vi "MK210_Query.vi"(7 "String":string, 8 "error in (no error)":errorcluster, 9 "Delay Time (s) 2":dbl=0.5, 10 "Delay Time (s)":dbl=0.5, 11 "DriverConnect in":T1) -> (0 "error out":errorcluster, 3 "DriverConnect out":T1, 4 "String from device out":string)   [LabVIEW 2018]
uses:
  MOKO_LabViewLibrary/MokoLowLevel/MokoLowLovelControl/MLLC_ConnectCluster.ctl
  MOKO_LabViewLibrary/MokoLowLevel/MokoLowLovelControl/MLLC_InterfaceType.ctl
  MOKO_LabViewLibrary/MokoLowLevel/MokoLowLovelControl/MLLC_OpenedSession.ctl
  MOKO_LabViewLibrary/MokoLowLevel/MokoLowLovelControl/MLLC_InterfaceSettings.ctl
  MOKO_LabViewLibrary/MokoLowLevel/MokoLowLovelControl/MLLC_InterfaceKind.ctl
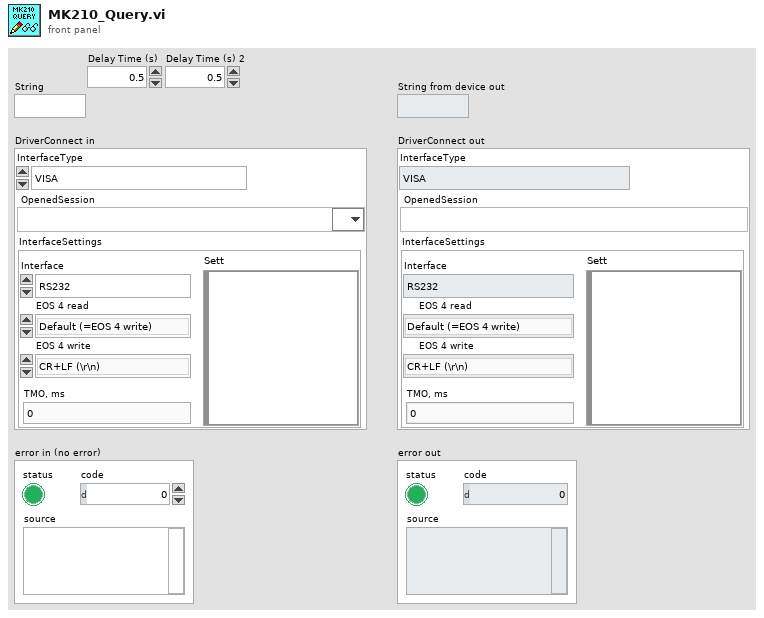
[diagram p1: front panel]
types:
  T1 = typedef "MLLC_ConnectCluster.ctl" = cluster{"InterfaceType":T2, "OpenedSession":T3, "InterfaceSettings":T4}
  T2 = typedef "MLLC_InterfaceType.ctl" = enum16{"VISA", "Prologix USB-GPIB"}
  T3 = typedef "MLLC_OpenedSession.ctl" = refnum<visa-resource-name>
  T4 = typedef "MLLC_InterfaceSettings.ctl" = cluster{"Interface":T5, "EOS 4 read":enum16{"Default (=EOS 4 write)", "CR (\\r)", "LF (\\n)", "None"}, "EOS 4 write":enum16{"CR+LF (\\r\\n)", "CR (\\r)", "LF (\\n)", "None"}, "TMO, ms":i32, "Sett":variant}
  T5 = typedef "MLLC_InterfaceKind.ctl" = enum16{"RS232", "GPIB", "USB", "Ethernet", "another"}
  T6 = typedef "MLLC_Error.ctl" = errorcluster
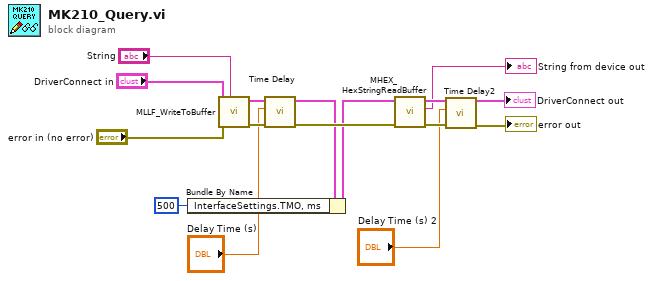
[diagram p0: block diagram]
diagram:
  n1 = call "MLLF_WriteToBuffer.vi"("String"="String", "error in"="error in (no error)", "DriverConnect in"="DriverConnect in") -> ("error out"=w12:T6, "DriverConnect out"=w6:T1)  [unwired: 5 in]
  n2 = Bundle By Name(cluster=w6, "InterfaceSettings.TMO, ms"=500) -> (w5:T1)
  n3 = call "Time Delay"("error in (no error)"=w12, "Delay Time (s)"="Delay Time (s)") -> ("error out"=w13:errorcluster)  [unwired: 9 in]
  n4 = call "MHEX_HexStringReadBuffer.vi"("error in"=w13, "DriverConnect in"=w5) -> ("error out"=w8:T6, "String from device out"=→"String from device out":string, "DriverConnect out"=→"DriverConnect out":T1)  [unwired: 6 in, 1 out]
  n5 = call "Time Delay2"("error in (no error)"=w8, "Delay Time (s)"="Delay Time (s) 2") -> ("error out"=→"error out":errorcluster)  [unwired: 9 in]
